vi "IMAQ forward movie.vi"(0 "Forwarded Phase":T1=refnum, 1 "n_grid":i32=300, 2 "Source Intensity":dbl[][](array[numeric])=array300x300[90000 elements], 5 "Forwarded Intensity":T1=refnum, 7 "error in (no error)":errorcluster, 9 "size_grid":dbl=0.001776, 11 "lambda":dbl=1.054e-06, 12 "Forward Distance":dbl=0.004106463878326996, 13 "Source Phase":sgl[][](array[numeric])=array300x300[90000 elements] format="%.2f") -> (15 "error out":errorcluster)   [LabVIEW 2012, in "LightPipes.lvlib"]
uses:
  LightPipes.lvlib
  <vilib>/vision/Image Controls.llb/IMAQ Image.ctl
panel:
  out "size(s)":i32[](array[numeric])=[300, 300]
  out "Forwarded Phase":T1(plugin-control)
  out "Forwared Int":T1(plugin-control)
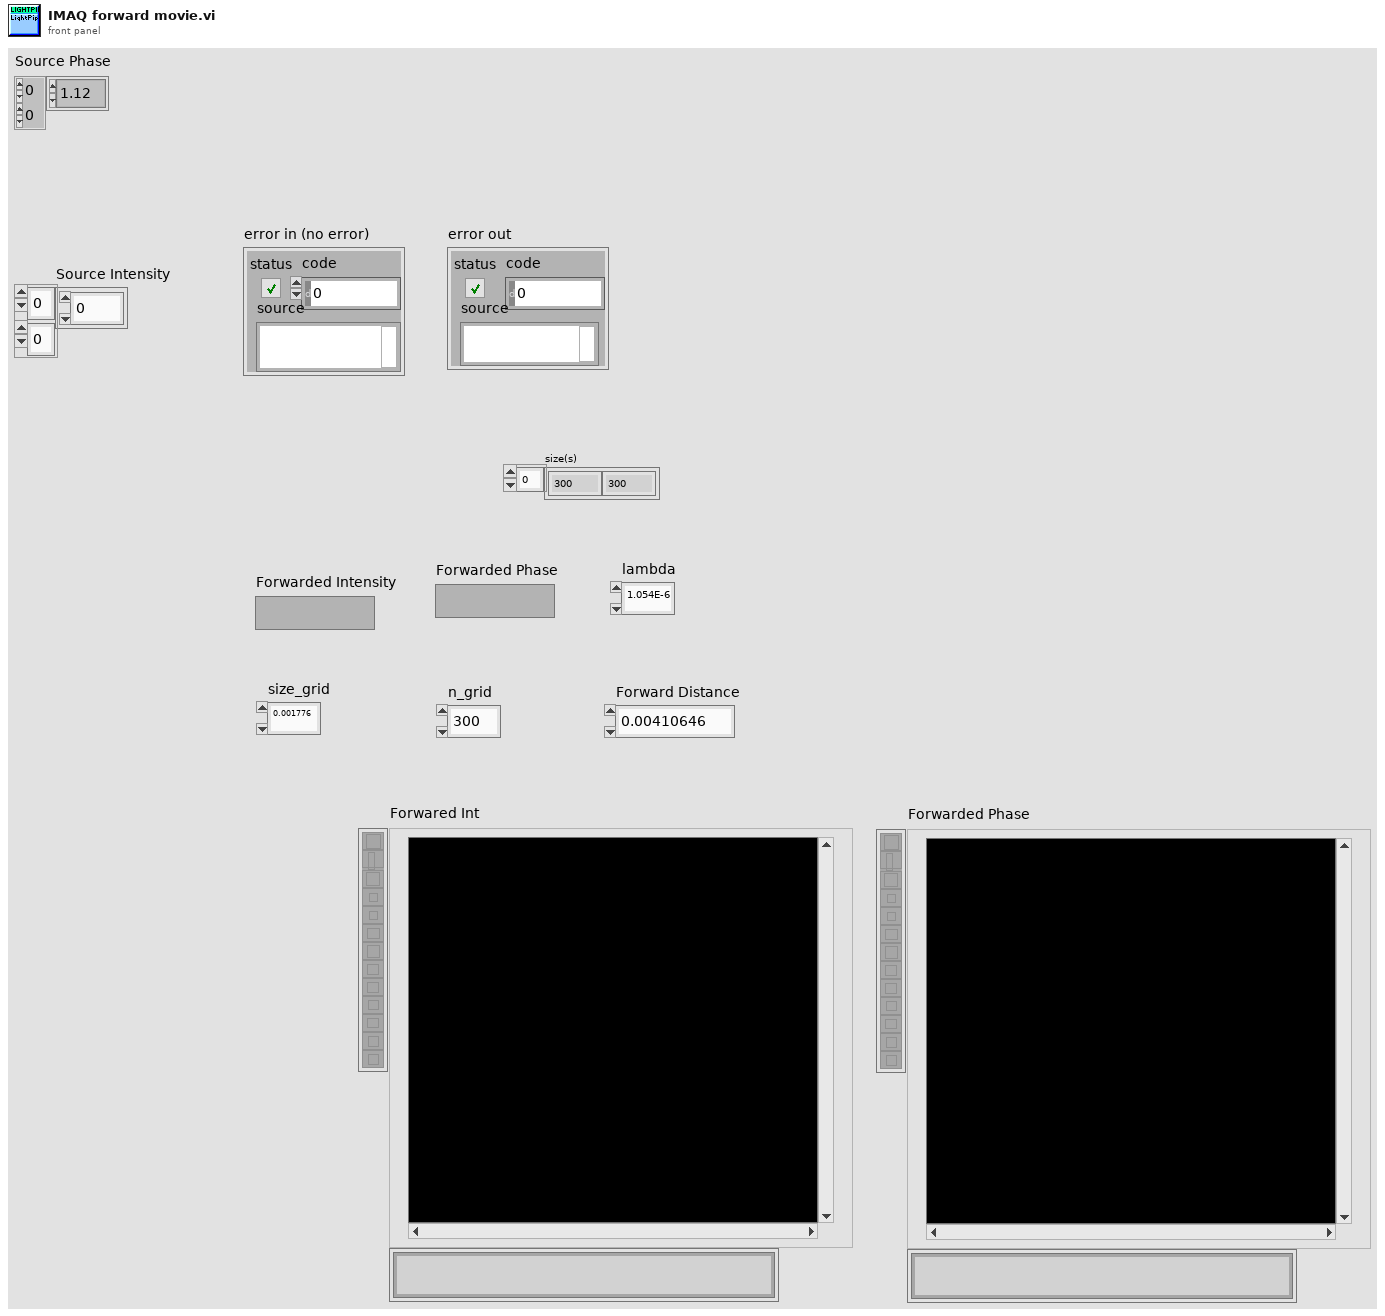
[diagram p1: front panel]
types:
  T1 = typedef "IMAQ Image.ctl" = refnum<image>
  T2 = cluster{"n_grid":i32, "@dummy control@":i8, "@dummy control@":i8, "@dummy control@":i8, "@dummy control@":i8, "size":dbl, "lambda":dbl, "int1":i32, "int2":i32, "int3":i32, "@dummy control@":i8, "@dummy control@":i8, "@dummy control@":i8, "@dummy control@":i8, "double1":dbl, "double2":dbl, "double3":dbl, "real":u32, "imaginary":u32}
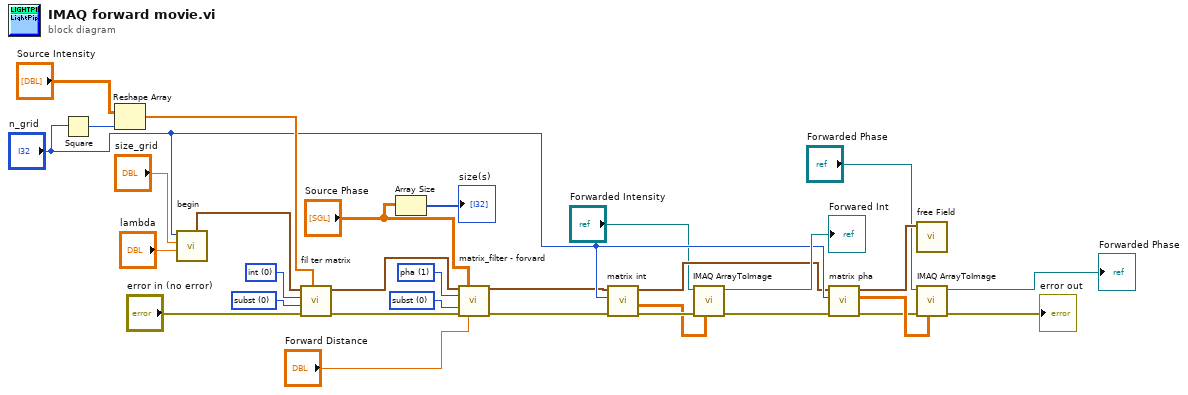
[diagram p0: block diagram]
diagram:
  w22 = i16 0 items=["subst", "mult"] ("multiplication/ substitution")
  w23 = i16 1 items=["int", "pha"] ("intensity / phase")
  w18 = i16 0 items=["int", "pha"] ("intensity / phase")
  w19 = i16 0 items=["subst", "mult"] ("multiplication/ substitution")
  n1 = Square(x="n_grid") -> (x^2=w27:i32)
  n2 = Reshape Array "Reshape Array"("Source Intensity", w27) -> (w28:dbl[])
  n3 = call "begin.vi"("lambda"="lambda", "size_grid"="size_grid", "n_grid"="n_grid") -> ("field out"=w21:T2)  [unwired: 8 in]
  n4 = call "fil ter matrix.vi"("matrix"=w28, "error in (no error)"="error in (no error)", "multiplication/ substitution"=w19, "intensity / phase"=w18, "field"=w21) -> ("error out"=w6:errorcluster, "field out"=w20:T2)  [unwired: 4 in, 1 out]
  n5 = Array Size(array="Source Phase") -> (size(s)=→"size(s)":i32[])
  n6 = call "matrix_filter - forvard.vi"("field"=w20, "matrix in"="Source Phase", "intensity/phase"=w23, "multiplication/substitution"=w22, "error in (no error)"=w6, "forward distance"="Forward Distance") -> ("field out"=w17:T2, "error out"=w13:errorcluster)  [unwired: 8 in]
  n7 = call "matrix int.vi"("error in (no error)"=w13, "n_grid"="n_grid", "field"=w17) -> ("error out"=w11:errorcluster, "matrix out 2D"=w1:dbl[][], "field out"=w16:T2)  [unwired: 6 in]
  n8 = call "IMAQ ArrayToImage"("Image Pixels (Float)"=w1, "error in (no error)"=w11, "Image"="Forwarded Intensity") -> ("error out"=w9:errorcluster, "Image Out"=→"Forwared Int":T1)  [unwired: 7 in]
  n9 = call "matrix pha.vi"("error in (no error)"=w9, "n_grid"="n_grid", "field"=w16) -> ("error out"=w10:errorcluster, "matrix out 2D"=w14:dbl[][], "field out"=w31:T2)  [unwired: 6 in]
  n10 = call "free Field.vi"("field"=w31) -> ()  [unwired: 10 in, 1 out]
  n11 = call "IMAQ ArrayToImage"("Image Pixels (Float)"=w14, "error in (no error)"=w10, "Image"="Forwarded Phase") -> ("error out"=→"error out":errorcluster, "Image Out"=→"Forwarded Phase":T1)  [unwired: 7 in]
